vi "Actor Core.vi"(8 "error in":errorcluster, 11 "Nested in":refnum<class "Coffee Actor.lvclass">) -> (0 "error out":errorcluster, 3 "Actor out":refnum<class "Actor.lvclass">)   [LabVIEW 2020, in "Coffee Actor.lvlib" / "Coffee Actor.lvclass"]
doc: "(<B>Filename</B>: Actor Framework.lvlib:Actor.lvclass:Actor Core.vi)\n\nReceives messages to the actor, reacts to them, and initiates any error handling that may shut the actor down.\n\nDescendant classes may override this VI to append parallel tasks for the actor to complete while it handles messages. Overrides use the Call Parent Method node."
uses:
  Coffee Actor.lvclass
  C:/Program Files/National Instruments/LabVIEW 2020/vi.lib/ActorFramework/Actor/Actor.lvclass
  <vilib>/ActorFramework/Actor/Actor.lvclass
  <vilib>/ActorFramework/Actor/Actor.lvclass/Actor.ctl
  <vilib>/ActorFramework/Message Enqueuer/Message Enqueuer.lvclass/Message Enqueuer.ctl
  Coffee Actor.lvclass/Coffee Actor.ctl
  <vilib>/ActorFramework/Message Enqueuer/Init from Existing Queue.vi
  <vilib>/ActorFramework/Message Enqueuer/Enqueue.vi
  <vilib>/ActorFramework/Stop Msg/Stop Msg.lvclass
  C:/Program Files/National Instruments/LabVIEW 2020/vi.lib/ActorFramework/Message/Message.lvclass
  <vilib>/ActorFramework/Message Priority Queue/Priority Enqueue.vi
  <vilib>/ActorFramework/Message Enqueuer/Message Enqueuer.lvclass
  C:/Users/deLili/Desktop/UDLSB IET/701/Instrumentacion Virtual/Fork/Maquina-2do-parcial/Coffee Actor/Coffee Actor.lvclass
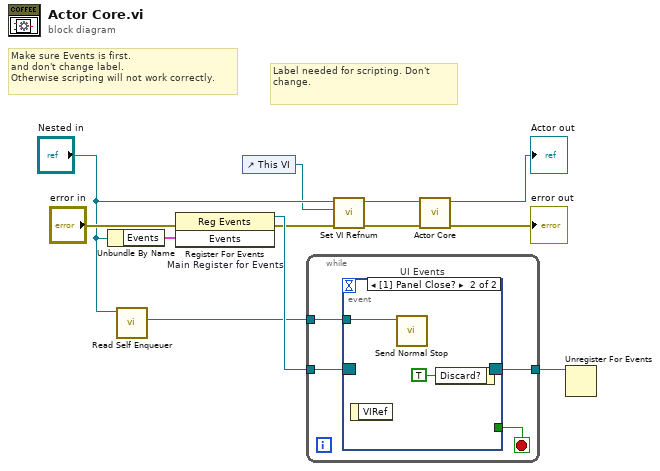
[diagram p0: block diagram]
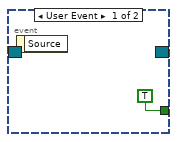
[diagram p2: hidden frame]
diagram:
  # "Label needed for scripting. Don't change."
  # "Make sure Events is first.\nand don't change label.\nOtherwise scripting will not work correctly."
  n1 = Unbundle By Name("Nested in") -> ("Events"=w9:cluster{"Stop":refnum<user-event>})
  n2 = call <vilib>:"Read Self Enqueuer.vi"("Actor"="Nested in") -> ("Self Enqueuer"=w7:refnum<class "Message Enqueuer.lvclass">)  [unwired: 10 in]
  n3 = register-events "Main Register for Events"(error in="error in", w9) -> (reference out=w10:refnum<event-registration>, error out=w3:errorcluster)  [unwired: 1 in]
  n4 = control-ref of="This VI"() -> (w1:refnum<vi>)
  n5 = while {
    tunnel: w10 -> [w16]
    tunnel: [w14] -> w8
    tunnel: w7 -> [w13]
    stop <- w15 stop-if-true
    n6 = event "UI Events" shown="[1] Panel Close?" {
      selector: w16 -> [_ _]
      dyn-events: [_ _] -> w14
      timeout: _ -> [_ _]
      tunnel: [TRUE _] -> w15
      tunnel: w13 -> [_ w18]
      event User Event {
        n7 = event-data() -> ()  [unwired: 1 in, 1 out]
      }
      event Panel Close? {
        n8 = event-data() -> ()  [unwired: 1 in, 1 out]
        n9 = call <vilib>:"Send Normal Stop.vi"("Message Enqueuer"=w18) -> ()  [unwired: 10 in, 1 out]
        n10 = event-data("Discard?"=TRUE) -> ()  [unwired: 1 in, 1 out]
      }
    }
  }
  n11 = call "Set VI Refnum.vi"("error in (no error)"=w3, "VI Refnum"=w1, "Coffee Actor in"="Nested in") -> ("error out"=w2:errorcluster, "Coffee Actor out"=w4:refnum<class "Coffee Actor.lvclass">)  [unwired: 7 in]
  n12 = call-parent "Actor Core.vi"("error in"=w2, "Actor in"=w4) -> ("error out"=→"error out":errorcluster, "Actor out"=→"Actor out":refnum<class "Actor.lvclass">)  [unwired: 8 in]
  n13 = Unregister For Events(event registration refnum=w8) -> ()  [unwired: 1 in, 1 out]
